vi "FloatApprox (Array).vi"(4 "y":dbl[](array[numeric]), 5 "x":dbl[](array[numeric])) -> (1 "x ~ y?":bool)   [LabVIEW 2016, in "Instrument.OxfordVRM.lvclass"]
doc: "Use to compare floating point numbers. This will check if two numbers are the same to 6 decimal places. Edit block diagram to change tolerance."
uses:
  Instrument.OxfordVRM.lvclass
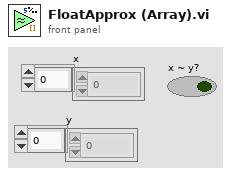
[diagram p1: front panel]
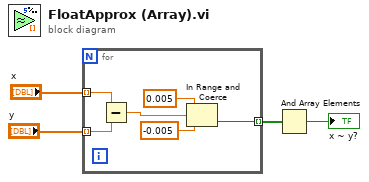
[diagram p0: block diagram]
diagram:
  n1 = for {
    tunnel: [w10] -> w4 mode=indexing
    tunnel: "y" -> [w9] mode=indexing
    tunnel: "x" -> [w8] mode=indexing
    n2 = Subtract(x=w8, y=w9) -> (x-y=w7:dbl)
    n3 = In Range and Coerce(upper limit=0.005, x=w7, lower limit=-0.005 ("upper limit")) -> (In Range?=w10:bool)  [unwired: 1 out]
  }
  n4 = And Array Elements(Boolean array=w4) -> (logical AND=→"x ~ y?":bool)
